vi "disconnect.vi"(8 "error in (no error)":errorcluster, 11 "comic_class in":refnum<class "comic_class.lvclass">) -> (0 "error out":errorcluster, 3 "comic_class out":refnum<class "comic_class.lvclass">)   [LabVIEW 2024, in "comic_class.lvclass"]
uses:
  comic_class.lvclass
  comic_class.lvclass/comic_class.ctl
  <vilib>/httpClient/LabVIEWHTTPClient.lvlib
  <vilib>/httpClient/ClientHandle.ctl
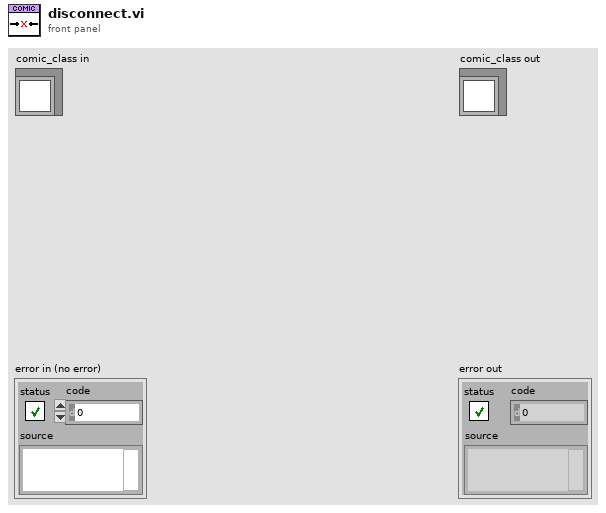
[diagram p1: front panel]
types:
  T1 = typedef "LabVIEWHTTPClient.lvlib/ClientHandle.ctl" = refnum<k1>
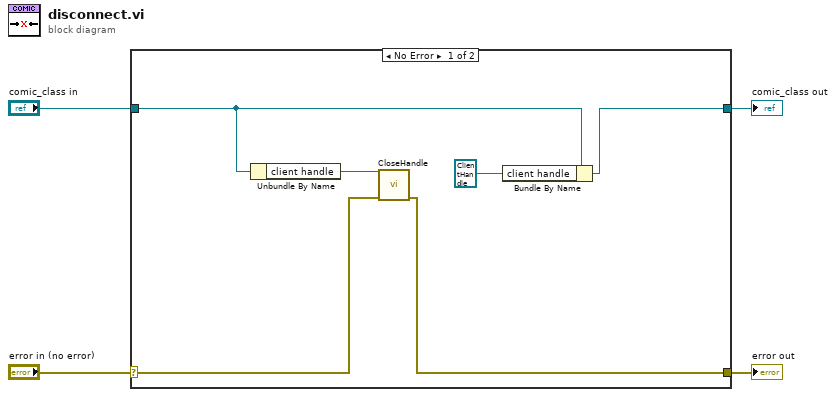
[diagram p0: block diagram]
diagram:
  n1 = case shown="No Error" "error in (no error)" {
    selector: "error in (no error)" -> [w6 w12]
    tunnel: [w5 w12] -> w3
    tunnel: [w8 w11] -> w1
    tunnel: "comic_class in" -> [w7 w11]
    frame No Error {
      n2 = Unbundle By Name(w7) -> ("client handle"=w10:T1)
      n3 = call <vilib>:"CloseHandle.vi"("client handle"=w10, "error in (no error)"=w6) -> ("error out"=w5:errorcluster)  [unwired: 13 in]
      n4 = Bundle By Name(cluster=w7, "client handle"=T1 refnum) -> (w8:refnum<class "comic_class.lvclass">)
    }
    frame Error {
    }
  }
  "error out" <- w3
  "comic_class out" <- w1
